vi "Safeties_2020_Build_Season.vi"   [LabVIEW 2019]
uses:
  Globals/Flywheel_Globals.vi
  Globals/Turret_Globals.vi
  Globals/Drive_Globals.vi
  Globals/Intake_Globals.vi
  Globals/Magazine_Globals.vi
  Globals/Control_Panel_Globals.vi
  Globals/Climb_Globals.vi
  <vilib>/Rock Robotics/WPI/ThirdParty/Phoenix-LabVIEW/Motor Controller/Get/CTRE_Phoenix_MotorController_IntegratedSensorData_TalonFX.vi
  <vilib>/Rock Robotics/WPI/ThirdParty/Phoenix-LabVIEW/Motor Controller/Get/CTRE_Phoenix_MotorController_GetSupplyAndStatorCurrent_Enhanced.vi
  <vilib>/Rock Robotics/Network Tables/NT Write Boolean.vi
types:
  T1 = typedef "WPI_MotorControlDeviceRef.ctl" = cluster{"DeviceStatus":errorcluster, "Type":T2, "PWM":cluster{"PWM Channel":T3, "DeadBand":T4}, "CAN":cluster{"Device Number":u8, "SetOutput VI Ref":variant, "GetOutput VI Ref":variant, "Enable VI Ref":variant, "Disable VI Ref":variant, "Data":variant}, "Invert":bool, "DIO PWM":cluster{"PWM \"Enable\" Channel":T3, "DIOChannel":T5, "PWM Rate":dbl}}
  T2 = typedef "WPI_MotorControlType.ctl" = enum16{"PWM", "CAN", "DIO PWM"}
  T3 = typedef "FPGA_DIOPWMChannel.ctl" = enum8{"PWM 0", "PWM 1", "PWM 2", "PWM 3", "PWM 4", "PWM 5", "PWM 6", "PWM 7", "PWM 8", "PWM 9", "PWM MXP 0", "PWM MXP 1", "PWM MXP 2", "PWM MXP 3", "PWM MXP 4", "PWM MXP 5", "PWM MXP 6", "PWM MXP 7", "PWM MXP 8", "PWM MXP 9", "Invalid"}
  T4 = typedef "WPI_PWMDeadband.ctl" = cluster{"Name":string, "maxPositivePwm":i32, "minPositivePwm":i32, "centerPwm":i32, "maxNegativePwm":i32, "minNegativePwm":i32, "angularRange":u16}
  T5 = typedef "FPGA_DIOChannel.ctl" = enum8{"DIO 0", "DIO 1", "DIO 2", "DIO 3", "DIO 4", "DIO 5", "DIO 6", "DIO 7", "DIO 8", "DIO 9", "DIO MXP 0", "DIO MXP 1", "DIO MXP 2", "DIO MXP 3", "DIO MXP 4", "DIO MXP 5", "DIO MXP 6", "DIO MXP 7", "DIO MXP 8", "DIO MXP 9", "DIO MXP 10", "DIO MXP 11", "DIO MXP 12", "DIO MXP 13", "DIO MXP 14", "DIO MXP 15", "SPI Port CS1", "SPI Port CS2", "SPI Port CS3", "SPI Port MISO", "SPI Port MOSI", "Invalid"}
  T6 = typedef "CTRE_PigeonIMU_DeviceRef.ctl" = cluster{"DeviceStatus":errorcluster, "Device Number":u8, "Type":T7, "Device ID":u32, "Handle":u64, "UsageFrame":u32, "Library Path":path}
  T7 = typedef "CTRE_PigeonIMU_ConnectionType.ctl" = u32
  T8 = typedef "WPI_AnalogChannelDevRef.ctl" = cluster{"DevStatus":errorcluster, "Analog Channel":T9}
  T9 = typedef "FPGA_AIChannel.ctl" = enum8{"AI 0", "AI 1", "AI 2", "AI 3", "AI MXP 0", "AI MXP 1", "AI MXP 2", "AI MXP 3", "Invalid"}
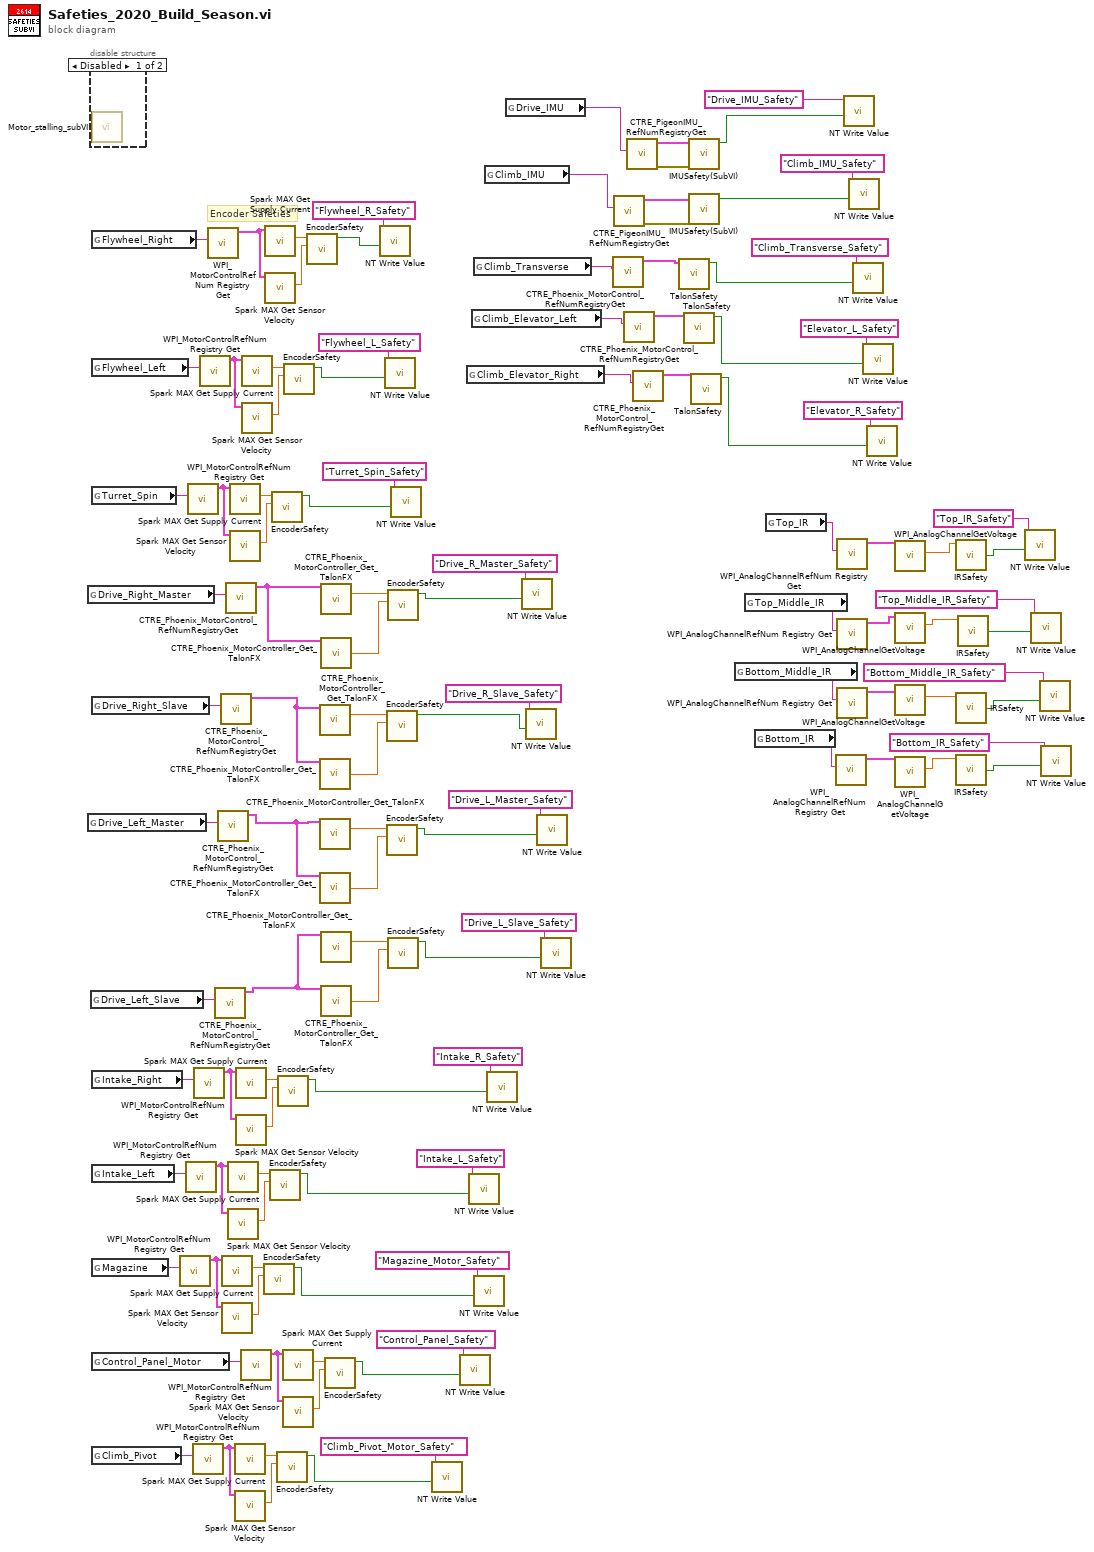
[diagram p0: block diagram]
diagram:
  # "Encoder Safeties"
  n1 = global read "Drive_Globals.vi" "Drive_Right_Master"() -> (w89:string)
  n2 = global read "Drive_Globals.vi" "Drive_Left_Master"() -> (w87:string)
  n3 = disable-structure shown="Disabled" {
    frame Disabled {
      n4 = call "Motor_stalling_subVI.vi"() -> ()  [unwired: 11 in, 1 out]
    }
    frame Enabled {
    }
  }
  n5 = global read "Drive_Globals.vi" "Drive_Left_Slave"() -> (w86:string)
  n6 = global read "Flywheel_Globals.vi" "Flywheel_Right"() -> (w114:string)
  n7 = global read "Flywheel_Globals.vi" "Flywheel_Left"() -> (w108:string)
  n8 = global read "Turret_Globals.vi" "Turret_Spin"() -> (w95:string)
  n9 = global read "Drive_Globals.vi" "Drive_Right_Slave"() -> (w88:string)
  n10 = global read "Intake_Globals.vi" "Intake_Right"() -> (w94:string)
  n11 = global read "Intake_Globals.vi" "Intake_Left"() -> (w93:string)
  n12 = global read "Magazine_Globals.vi" "Magazine"() -> (w92:string)
  n13 = global read "Control_Panel_Globals.vi" "Control_Panel_Motor"() -> (w91:string)
  n14 = global read "Climb_Globals.vi" "Climb_Pivot"() -> (w90:string)
  n15 = call <vilib>:"WPI_MotorControlRefNum Registry Get.vi"("refnum name"=w92) -> ("MotorControlDevRef"=w75:T1)  [unwired: 9 in, 1 out]
  n16 = call <vilib>:"WPI_MotorControlRefNum Registry Get.vi"("refnum name"=w93) -> ("MotorControlDevRef"=w77:T1)  [unwired: 9 in, 1 out]
  n17 = call <vilib>:"WPI_MotorControlRefNum Registry Get.vi"("refnum name"=w95) -> ("MotorControlDevRef"=w78:T1)  [unwired: 9 in, 1 out]
  n18 = call <vilib>:"WPI_MotorControlRefNum Registry Get.vi"("refnum name"=w90) -> ("MotorControlDevRef"=w73:T1)  [unwired: 9 in, 1 out]
  n19 = call <vilib>:"WPI_MotorControlRefNum Registry Get.vi"("refnum name"=w94) -> ("MotorControlDevRef"=w76:T1)  [unwired: 9 in, 1 out]
  n20 = call <vilib>:"WPI_MotorControlRefNum Registry Get.vi"("refnum name"=w108) -> ("MotorControlDevRef"=w79:T1)  [unwired: 9 in, 1 out]
  n21 = call <vilib>:"WPI_MotorControlRefNum Registry Get.vi"("refnum name"=w114) -> ("MotorControlDevRef"=w113:T1)  [unwired: 9 in, 1 out]
  n22 = call <vilib>:"CTRE_Phoenix_MotorControl_RefNumRegistryGet.vi"("refnum name"=w86) -> ("PhoenixMotorControlDevRef"=w58:T1)  [unwired: 9 in, 1 out]
  n23 = call <vilib>:"CTRE_Phoenix_MotorControl_RefNumRegistryGet.vi"("refnum name"=w87) -> ("PhoenixMotorControlDevRef"=w61:T1)  [unwired: 9 in, 1 out]
  n24 = call <vilib>:"CTRE_Phoenix_MotorControl_RefNumRegistryGet.vi"("refnum name"=w88) -> ("PhoenixMotorControlDevRef"=w64:T1)  [unwired: 9 in, 1 out]
  n25 = call <vilib>:"Spark MAX Get Supply Current.vi"("MotorControlDevRef in"=w75) -> ("Current"=w100:dbl)  [unwired: 7 in, 3 out]
  n26 = call <vilib>:"Spark MAX Get Sensor Velocity.vi"("MotorControlDevRef in"=w75) -> ("Sensor Velocity"=w101:dbl)  [unwired: 7 in, 3 out]
  n27 = call <vilib>:"CTRE_Phoenix_MotorControl_RefNumRegistryGet.vi"("refnum name"=w89) -> ("PhoenixMotorControlDevRef"=w69:T1)  [unwired: 9 in, 1 out]
  n28 = call <vilib>:"Spark MAX Get Supply Current.vi"("MotorControlDevRef in"=w77) -> ("Current"=w102:dbl)  [unwired: 7 in, 3 out]
  n29 = call <vilib>:"Spark MAX Get Sensor Velocity.vi"("MotorControlDevRef in"=w77) -> ("Sensor Velocity"=w103:dbl)  [unwired: 7 in, 3 out]
  n30 = call <vilib>:"Spark MAX Get Supply Current.vi"("MotorControlDevRef in"=w78) -> ("Current"=w106:dbl)  [unwired: 7 in, 3 out]
  n31 = call <vilib>:"Spark MAX Get Sensor Velocity.vi"("MotorControlDevRef in"=w78) -> ("Sensor Velocity"=w107:dbl)  [unwired: 7 in, 3 out]
  n32 = call <vilib>:"Spark MAX Get Supply Current.vi"("MotorControlDevRef in"=w73) -> ("Current"=w96:dbl)  [unwired: 7 in, 3 out]
  n33 = call <vilib>:"Spark MAX Get Sensor Velocity.vi"("MotorControlDevRef in"=w73) -> ("Sensor Velocity"=w97:dbl)  [unwired: 7 in, 3 out]
  n34 = call <vilib>:"Spark MAX Get Supply Current.vi"("MotorControlDevRef in"=w76) -> ("Current"=w104:dbl)  [unwired: 7 in, 3 out]
  n35 = call <vilib>:"Spark MAX Get Sensor Velocity.vi"("MotorControlDevRef in"=w76) -> ("Sensor Velocity"=w105:dbl)  [unwired: 7 in, 3 out]
  n36 = call <vilib>:"WPI_MotorControlRefNum Registry Get.vi"("refnum name"=w91) -> ("MotorControlDevRef"=w74:T1)  [unwired: 9 in, 1 out]
  n37 = call <vilib>:"Spark MAX Get Supply Current.vi"("MotorControlDevRef in"=w79) -> ("Current"=w109:dbl)  [unwired: 7 in, 3 out]
  n38 = call <vilib>:"Spark MAX Get Sensor Velocity.vi"("MotorControlDevRef in"=w79) -> ("Sensor Velocity"=w110:dbl)  [unwired: 7 in, 3 out]
  n39 = call "EncoderSafety.vi"("Motor Velocity"=w101, "Motor Current"=w100) -> ("Encoder_Dead?"=w32:bool)  [unwired: 8 in]
  n40 = call <vilib>:"Spark MAX Get Supply Current.vi"("MotorControlDevRef in"=w113) -> ("Current"=w111:dbl)  [unwired: 7 in, 3 out]
  n41 = call <vilib>:"Spark MAX Get Sensor Velocity.vi"("MotorControlDevRef in"=w113) -> ("Sensor Velocity"=w112:dbl)  [unwired: 7 in, 3 out]
  n42 = call "EncoderSafety.vi"("Motor Velocity"=w103, "Motor Current"=w102) -> ("Encoder_Dead?"=w33:bool)  [unwired: 8 in]
  n43 = call "EncoderSafety.vi"("Motor Velocity"=w107, "Motor Current"=w106) -> ("Encoder_Dead?"=w39:bool)  [unwired: 8 in]
  n44 = call "EncoderSafety.vi"("Motor Velocity"=w97, "Motor Current"=w96) -> ("Encoder_Dead?"=w30:bool)  [unwired: 8 in]
  n45 = call "EncoderSafety.vi"("Motor Velocity"=w105, "Motor Current"=w104) -> ("Encoder_Dead?"=w34:bool)  [unwired: 8 in]
  n46 = call <vilib>:"Spark MAX Get Supply Current.vi"("MotorControlDevRef in"=w74) -> ("Current"=w98:dbl)  [unwired: 7 in, 3 out]
  n47 = call <vilib>:"Spark MAX Get Sensor Velocity.vi"("MotorControlDevRef in"=w74) -> ("Sensor Velocity"=w99:dbl)  [unwired: 7 in, 3 out]
  n48 = call "EncoderSafety.vi"("Motor Velocity"=w110, "Motor Current"=w109) -> ("Encoder_Dead?"=w40:bool)  [unwired: 8 in]
  n49 = call "EncoderSafety.vi"("Motor Velocity"=w112, "Motor Current"=w111) -> ("Encoder_Dead?"=w57:bool)  [unwired: 8 in]
  n50 = call-poly <vilib>:"CTRE_Phoenix_MotorController_Get_TalonFX.vi"("PhoenixMotorControlDevRef"=w64) -> ("Supply Current"=w66:dbl)  [unwired: 11 in, 3 out]
  n51 = call-poly <vilib>:"CTRE_Phoenix_MotorController_Get_TalonFX.vi"("PhoenixMotorControlDevRef"=w64) -> ("Velocity"=w65:dbl)  [unwired: 10 in, 4 out]
  n52 = call-poly <vilib>:"CTRE_Phoenix_MotorController_Get_TalonFX.vi"("PhoenixMotorControlDevRef"=w61) -> ("Supply Current"=w63:dbl)  [unwired: 11 in, 3 out]
  n53 = call-poly <vilib>:"CTRE_Phoenix_MotorController_Get_TalonFX.vi"("PhoenixMotorControlDevRef"=w61) -> ("Velocity"=w62:dbl)  [unwired: 10 in, 4 out]
  n54 = call-poly <vilib>:"CTRE_Phoenix_MotorController_Get_TalonFX.vi"("PhoenixMotorControlDevRef"=w69) -> ("Supply Current"=w68:dbl)  [unwired: 11 in, 3 out]
  n55 = call-poly <vilib>:"CTRE_Phoenix_MotorController_Get_TalonFX.vi"("PhoenixMotorControlDevRef"=w69) -> ("Velocity"=w67:dbl)  [unwired: 10 in, 4 out]
  n56 = call-poly <vilib>:"CTRE_Phoenix_MotorController_Get_TalonFX.vi"("PhoenixMotorControlDevRef"=w58) -> ("Supply Current"=w60:dbl)  [unwired: 11 in, 3 out]
  n57 = call-poly <vilib>:"CTRE_Phoenix_MotorController_Get_TalonFX.vi"("PhoenixMotorControlDevRef"=w58) -> ("Velocity"=w59:dbl)  [unwired: 10 in, 4 out]
  n58 = call "EncoderSafety.vi"("Motor Velocity"=w99, "Motor Current"=w98) -> ("Encoder_Dead?"=w31:bool)  [unwired: 8 in]
  n59 = call-poly <vilib>:"NT Write Value.vi"("Boolean"=w57, "Name"="Flywheel_R_Safety") -> ()  [unwired: 9 in, 1 out]
  n60 = call-poly <vilib>:"NT Write Value.vi"("Boolean"=w40, "Name"="Flywheel_L_Safety") -> ()  [unwired: 9 in, 1 out]
  n61 = call "EncoderSafety.vi"("Motor Velocity"=w65, "Motor Current"=w66) -> ("Encoder_Dead?"=w37:bool)  [unwired: 8 in]
  n62 = call "EncoderSafety.vi"("Motor Velocity"=w62, "Motor Current"=w63) -> ("Encoder_Dead?"=w36:bool)  [unwired: 8 in]
  n63 = call "EncoderSafety.vi"("Motor Velocity"=w67, "Motor Current"=w68) -> ("Encoder_Dead?"=w38:bool)  [unwired: 8 in]
  n64 = call "EncoderSafety.vi"("Motor Velocity"=w59, "Motor Current"=w60) -> ("Encoder_Dead?"=w35:bool)  [unwired: 8 in]
  n65 = call-poly <vilib>:"NT Write Value.vi"("Boolean"=w39, "Name"="Turret_Spin_Safety") -> ()  [unwired: 9 in, 1 out]
  n66 = call-poly <vilib>:"NT Write Value.vi"("Boolean"=w30, "Name"="Climb_Pivot_Motor_Safety") -> ()  [unwired: 9 in, 1 out]
  n67 = call-poly <vilib>:"NT Write Value.vi"("Boolean"=w31, "Name"="Control_Panel_Safety") -> ()  [unwired: 9 in, 1 out]
  n68 = global read "Climb_Globals.vi" "Climb_Elevator_Right"() -> (w85:string)
  n69 = call-poly <vilib>:"NT Write Value.vi"("Boolean"=w33, "Name"="Intake_L_Safety") -> ()  [unwired: 9 in, 1 out]
  n70 = global read "Climb_Globals.vi" "Climb_Elevator_Left"() -> (w84:string)
  n71 = global read "Climb_Globals.vi" "Climb_Transverse"() -> (w83:string)
  n72 = call-poly <vilib>:"NT Write Value.vi"("Boolean"=w32, "Name"="Magazine_Motor_Safety") -> ()  [unwired: 9 in, 1 out]
  n73 = global read "Climb_Globals.vi" "Climb_IMU"() -> (w72:string)
  n74 = call-poly <vilib>:"NT Write Value.vi"("Boolean"=w34, "Name"="Intake_R_Safety") -> ()  [unwired: 9 in, 1 out]
  n75 = global read "Drive_Globals.vi" "Drive_IMU"() -> (w5:string)
  n76 = call-poly <vilib>:"NT Write Value.vi"("Boolean"=w38, "Name"="Drive_R_Master_Safety") -> ()  [unwired: 9 in, 1 out]
  n77 = call-poly <vilib>:"NT Write Value.vi"("Boolean"=w37, "Name"="Drive_R_Slave_Safety") -> ()  [unwired: 9 in, 1 out]
  n78 = call-poly <vilib>:"NT Write Value.vi"("Boolean"=w36, "Name"="Drive_L_Master_Safety") -> ()  [unwired: 9 in, 1 out]
  n79 = call-poly <vilib>:"NT Write Value.vi"("Boolean"=w35, "Name"="Drive_L_Slave_Safety") -> ()  [unwired: 9 in, 1 out]
  n80 = call <vilib>:"CTRE_Phoenix_MotorControl_RefNumRegistryGet.vi"("refnum name"=w83) -> ("PhoenixMotorControlDevRef"=w82:T1)  [unwired: 9 in, 1 out]
  n81 = call <vilib>:"CTRE_PigeonIMU_RefNumRegistryGet.vi"("refnum name"=w72) -> ("error out"=w71:errorcluster, "PigeonIMUDevRef"=w70:T6)  [unwired: 9 in]
  n82 = call <vilib>:"CTRE_Phoenix_MotorControl_RefNumRegistryGet.vi"("refnum name"=w84) -> ("PhoenixMotorControlDevRef"=w81:T1)  [unwired: 9 in, 1 out]
  n83 = call <vilib>:"CTRE_PigeonIMU_RefNumRegistryGet.vi"("refnum name"=w5) -> ("error out"=w3:errorcluster, "PigeonIMUDevRef"=w4:T6)  [unwired: 9 in]
  n84 = call <vilib>:"CTRE_Phoenix_MotorControl_RefNumRegistryGet.vi"("refnum name"=w85) -> ("PhoenixMotorControlDevRef"=w80:T1)  [unwired: 9 in, 1 out]
  n85 = call "TalonSafety.vi"("PhoenixMotorControlDevRef"=w82) -> ("Encoder_Dead?"=w28:bool)  [unwired: 10 in]
  n86 = call "TalonSafety.vi"("PhoenixMotorControlDevRef"=w81) -> ("Encoder_Dead?"=w27:bool)  [unwired: 10 in]
  n87 = call "IMUSafety(SubVI).vi"("error in (no error)"=w3, "PigeonIMUDevRef"=w4) -> ("Boolean"=w1:bool)  [unwired: 9 in]
  n88 = call "IMUSafety(SubVI).vi"("error in (no error)"=w71, "PigeonIMUDevRef"=w70) -> ("Boolean"=w29:bool)  [unwired: 9 in]
  n89 = call "TalonSafety.vi"("PhoenixMotorControlDevRef"=w80) -> ("Encoder_Dead?"=w26:bool)  [unwired: 10 in]
  n90 = global read "Magazine_Globals.vi" "Bottom_Middle_IR"() -> (w23:string)
  n91 = global read "Magazine_Globals.vi" "Top_Middle_IR"() -> (w24:string)
  n92 = global read "Magazine_Globals.vi" "Bottom_IR"() -> (w22:string)
  n93 = global read "Magazine_Globals.vi" "Top_IR"() -> (w25:string)
  n94 = call <vilib>:"WPI_AnalogChannelRefNum Registry Get.vi"("refnum name"=w22) -> ("AIDeviceRef"=w18:T8)  [unwired: 9 in, 1 out]
  n95 = call <vilib>:"WPI_AnalogChannelRefNum Registry Get.vi"("refnum name"=w25) -> ("AIDeviceRef"=w20:T8)  [unwired: 9 in, 1 out]
  n96 = call <vilib>:"WPI_AnalogChannelRefNum Registry Get.vi"("refnum name"=w24) -> ("AIDeviceRef"=w21:T8)  [unwired: 9 in, 1 out]
  n97 = call <vilib>:"WPI_AnalogChannelRefNum Registry Get.vi"("refnum name"=w23) -> ("AIDeviceRef"=w19:T8)  [unwired: 9 in, 1 out]
  n98 = call-poly <vilib>:"NT Write Value.vi"("Boolean"=w1, "Name"="Drive_IMU_Safety") -> ()  [unwired: 9 in, 1 out]
  n99 = call-poly <vilib>:"NT Write Value.vi"("Boolean"=w29, "Name"="Climb_IMU_Safety") -> ()  [unwired: 9 in, 1 out]
  n100 = call-poly <vilib>:"NT Write Value.vi"("Boolean"=w28, "Name"="Climb_Transverse_Safety") -> ()  [unwired: 9 in, 1 out]
  n101 = call-poly <vilib>:"NT Write Value.vi"("Boolean"=w27, "Name"="Elevator_L_Safety") -> ()  [unwired: 9 in, 1 out]
  n102 = call-poly <vilib>:"NT Write Value.vi"("Boolean"=w26, "Name"="Elevator_R_Safety") -> ()  [unwired: 9 in, 1 out]
  n103 = call <vilib>:"WPI_AnalogChannelGetVoltage.vi"("AIDeviceRef"=w20) -> ("Voltage"=w17:dbl)  [unwired: 8 in, 2 out]
  n104 = call <vilib>:"WPI_AnalogChannelGetVoltage.vi"("AIDeviceRef"=w21) -> ("Voltage"=w16:dbl)  [unwired: 8 in, 2 out]
  n105 = call <vilib>:"WPI_AnalogChannelGetVoltage.vi"("AIDeviceRef"=w19) -> ("Voltage"=w15:dbl)  [unwired: 8 in, 2 out]
  n106 = call <vilib>:"WPI_AnalogChannelGetVoltage.vi"("AIDeviceRef"=w18) -> ("Voltage"=w14:dbl)  [unwired: 8 in, 2 out]
  n107 = call "IRSafety.vi"("Voltage"=w17) -> ("Boolean"=w10:bool)  [unwired: 3 in]
  n108 = call "IRSafety.vi"("Voltage"=w15) -> ("Boolean"=w13:bool)  [unwired: 3 in]
  n109 = call "IRSafety.vi"("Voltage"=w14) -> ("Boolean"=w12:bool)  [unwired: 3 in]
  n110 = call "IRSafety.vi"("Voltage"=w16) -> ("Boolean"=w11:bool)  [unwired: 3 in]
  n111 = call-poly <vilib>:"NT Write Value.vi"("Boolean"=w10, "Name"="Top_IR_Safety") -> ()  [unwired: 9 in, 1 out]
  n112 = call-poly <vilib>:"NT Write Value.vi"("Boolean"=w11, "Name"="Top_Middle_IR_Safety") -> ()  [unwired: 9 in, 1 out]
  n113 = call-poly <vilib>:"NT Write Value.vi"("Boolean"=w13, "Name"="Bottom_Middle_IR_Safety") -> ()  [unwired: 9 in, 1 out]
  n114 = call-poly <vilib>:"NT Write Value.vi"("Boolean"=w12, "Name"="Bottom_IR_Safety") -> ()  [unwired: 9 in, 1 out]
